vi "Test cluster2json.vi"() -> ()   [LabVIEW 2011, in "JSON.lvlib"]
uses:
  JSON.lvlib
panel:
  out "error out":errorcluster
  out "JSON":string="{\n  \"String\": \"fdqfdqfdq ' \\\" \\\\\"\r  ,\"Bool\": false\r  ,\"acceleration\": 789.456789\r  ,\"Unsigned\": 532\r  ,\"Word\": 12\r  ,\"Titre tableau\": [1.250000,25.600000]\r  ,\"Acc components\": {\n  \"mean\": 45.000000\r  ,\"std\": 5.200000\r\n}\r\n}"
  in  "Cluster":T1={"String"="fdqfdqfdq ' \" \\", "Bool"=FALSE, "acceleration"=789.456789456, "Unsigned"=532, "Word"=12, "Titre tableau"=[1.25, 25.6], "Acc components"={"mean"=45.0, "std"=5.2}, "Autre tableau"=["aer", "re", "jkl; \"mfdqj"], "Array"=[]} {"acceleration" format="%#_100g"}
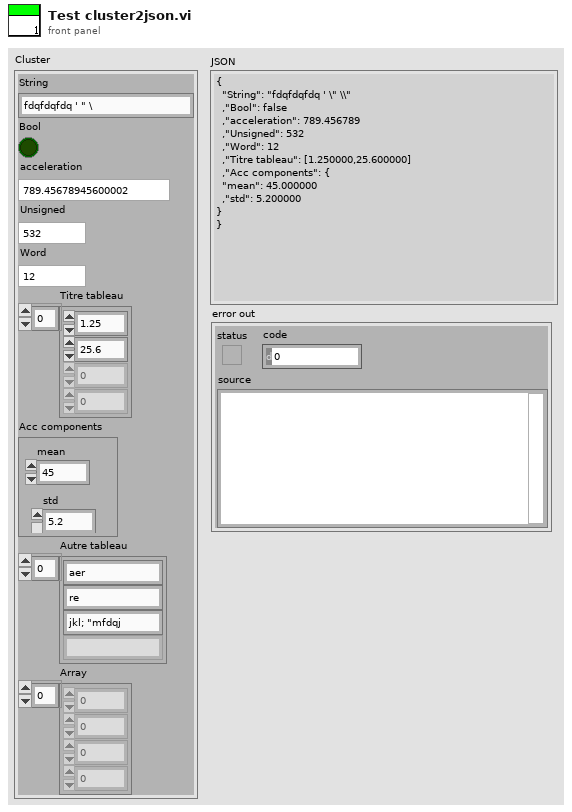
[diagram p1: front panel]
types:
  T1 = cluster{"String":string, "Bool":bool, "acceleration":dbl, "Unsigned":u16, "Word":i32, "Titre tableau":dbl[], "Acc components":cluster{"mean":dbl, "std":dbl}, "Autre tableau":string[], "Array":u32[]}
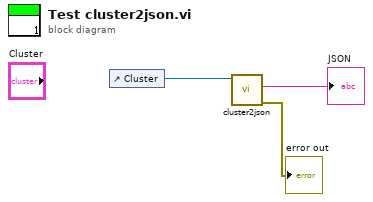
[diagram p0: block diagram]
diagram:
  n1 = control-ref of="Cluster"() -> (w3:refnum<vi>)
  n2 = call "cluster2json.vi"("Cluster Ref in"=w3) -> ("error out"=→"error out":errorcluster, "JSON"=→"JSON":string)  [unwired: 8 in, 1 out]
